vi "表格未开启时重启.vi"(8 "error in":errorcluster caption="错误in", 9 "worksheet name":string="ASDE", 10 "Path":path=path "D:/123.xls") -> (0 "error out":errorcluster caption="错误输出", 3 "表格是否打开":bool)   [LabVIEW 2014]
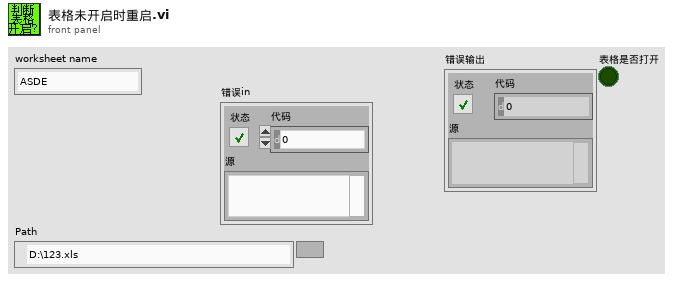
[diagram p1: front panel]
types:
  T1 = typedef "控件-Excel读写选项.ctl" = enum16{"打开表格", "新增sheet", "读取sheet指定位置数据", "读取sheet整个数据", "写入sheet整个数据", "写表头", "数据存到本机", "表格是否开启状态", "关闭表格"}
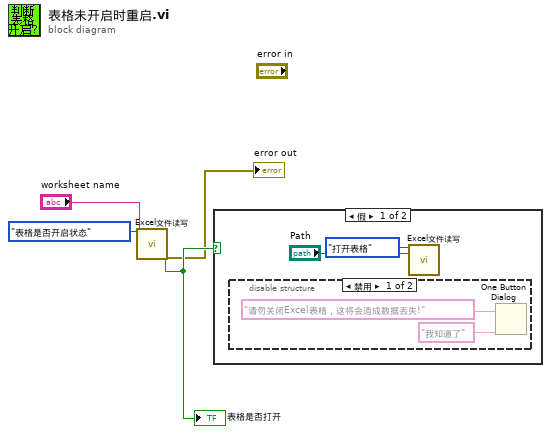
[diagram p0: block diagram]
diagram:
  n1 = call "Excel文件读写.vi"("选项"=控件-Excel读写选项."表格是否开启状态", "sheet name"="worksheet name") -> ("表格操作正常"=w3:bool, "error out"=→"error out":errorcluster)  [unwired: 15 in, 1 out]
  "表格是否打开" <- w3
  n2 = case shown="假" w3 {
    frame False {
      n3 = disable-structure shown="禁用" {
        frame Disabled {
          n4 = One Button Dialog(message="请勿关闭Excel表格，这将会造成数据丢失!" ("消息"), button name ("OK")="我知道了" ("按钮名称（“确定”）")) -> ()  [unwired: 1 out]
        }
        frame Enabled {
        }
      }
      n5 = call "Excel文件读写.vi"("选项"=控件-Excel读写选项."打开表格", "Path"="Path") -> ()  [unwired: 15 in, 3 out]
    }
    frame True {
    }
  }
